vi "CheckColision_1AsterNShoots.vi"(8 "Error In":errorcluster, 9 "ShootsInfo":cluster{"ShootData":T1, "Cluster":T2}[](array[cluster]), 10 "AsterData":T2, 11 "AsterObjectRef":refnum<vi>) -> (0 "Error Out":errorcluster, 1 "ShootsInfoOut":cluster{"ShootData":T1, "Cluster":T2}[](array[cluster]))   [LabVIEW 2017]
uses:
  HoldData/DataForColision.ctl
  ManRef_ShootData.ctl
  Asteroid/Asteroid_states.ctl
  Spaceship/Shoot/Shoot_states.ctl
  HoldData/HoldData_mods.ctl
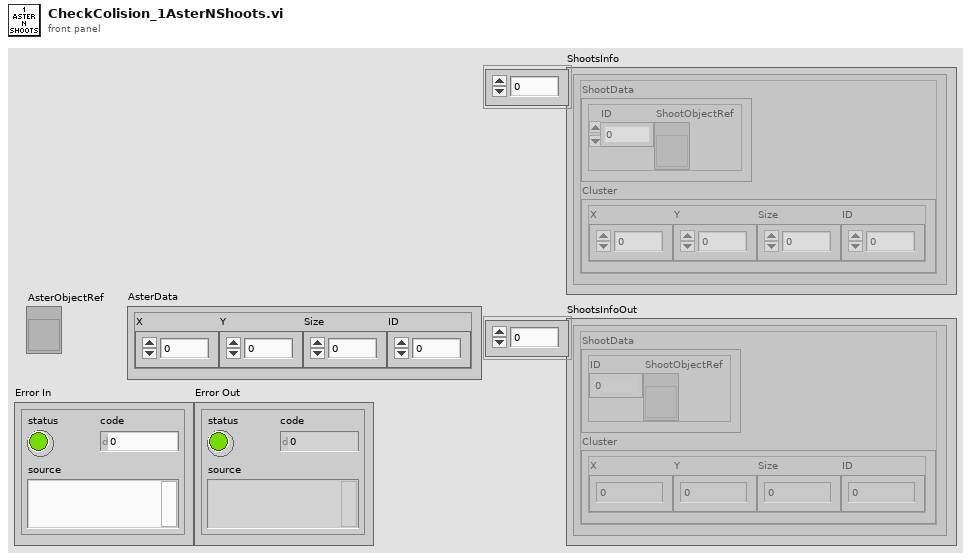
[diagram p1: front panel]
types:
  T1 = typedef "ManRef_ShootData.ctl" = cluster{"ID":i32, "ShootObjectRef":refnum<vi>}
  T2 = typedef "DataForColision.ctl" = cluster{"X":dbl, "Y":dbl, "Size":dbl, "ID":i32}
  T3 = typedef "HoldData_mods.ctl" = enum16{"Init", "NewAster", "UpdateAster", "RemoveAster", "GetAsterData", "NewShoot", "UpdateShoot", "RemoveShoot", "GetShootData", "End"}
  T4 = typedef "Shoot_states.ctl" = enum16{"Init", "Move", "Draw", "Destroy"}
  T5 = typedef "Asteroid_states.ctl" = enum16{"Init", "Move", "Split", "Draw", "Destroy"}
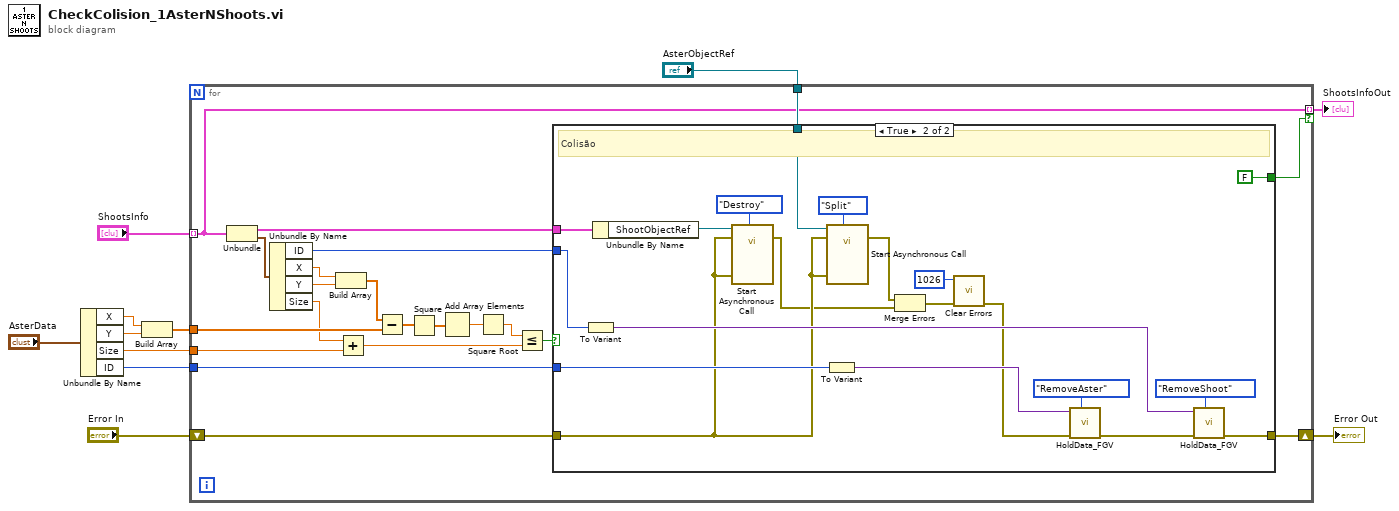
[diagram p0: block diagram]
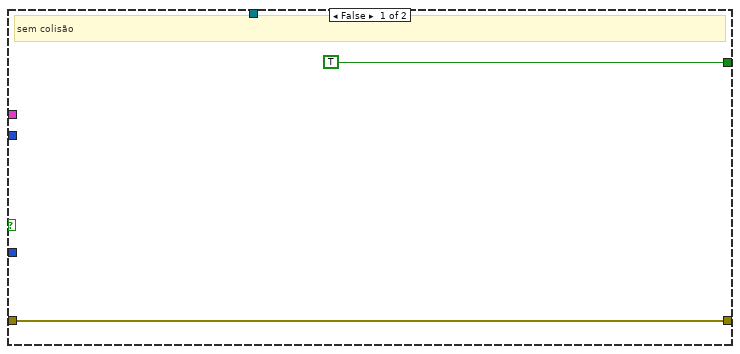
[diagram p2: hidden frame]
diagram:
  n1 = Unbundle By Name("AsterData") -> ("X"=w10:dbl, "Y"=w11:dbl, "Size"=w5:dbl, "ID"=w1:i32)
  n2 = Build Array(w10, w11) -> (w9:dbl[])
  n3 = for {
    tunnel: w5 -> [w16]
    tunnel: w9 -> [w29]
    shift-right: [w22] -> w7
    shift-left: "Error In" -> [w23]
    tunnel: "AsterObjectRef" -> [w21]
    tunnel: "ShootsInfo" -> [w18] mode=indexing
    tunnel: [w18] -> w2 mode=indexing if=w17
    tunnel: w1 -> [w13]
    n4 = Unbundle(w18) -> ("ShootData"=w20:T1, "Cluster"=w19:T2)
    n5 = Unbundle By Name(w19) -> ("ID"=w12:i32, "X"=w32:dbl, "Y"=w31:dbl, "Size"=w15:dbl)
    n6 = Build Array(w32, w31) -> (w30:dbl[])
    n7 = Add(x=w15, y=w16) -> (x+y=w14:dbl)
    n8 = Subtract(x=w30, y=w29) -> (x-y=w28:dbl[])
    n9 = Square(x=w28) -> (x^2=w27:dbl[])
    n10 = Add Array Elements(numeric array=w27) -> (sum=w26:dbl)
    n11 = Square Root(x=w26) -> (sqrt(x)=w25:dbl)
    n12 = Less Or Equal?(x=w25, y=w14) -> (x <= y?=w24:bool)
    n13 = case shown="True" w24 {
      tunnel: w20 -> [_ w54]
      tunnel: w23 -> [w34 w38]
      tunnel: [w34 w42] -> w22
      tunnel: w21 -> [_ w53]
      tunnel: [TRUE FALSE] -> w17
      tunnel: w13 -> [_ w47]
      tunnel: w12 -> [_ w45]
      frame False {
        # "sem colisão"
      }
      frame True {
        # "Colisão"
        n14 = To Variant(anything=w45) -> (Variant=w41:variant)
        n15 = Unbundle By Name(w54) -> ("ShootObjectRef"=w51:refnum<vi>)
        n16 = call-by-ref "Start Asynchronous Call"(reference=w51, error in=w38, "Shoot_states"=Shoot_states."Destroy", "error in"=w38) -> (error out=w37:errorcluster)  [unwired: 9 in, 2 out]
        n17 = call-by-ref "Start Asynchronous Call"(reference=w53, error in=w38, "Asteroid_states"=Asteroid_states."Split", "error in"=w38) -> (error out=w36:errorcluster)  [unwired: 9 in, 2 out]
        n18 = To Variant(anything=w47) -> (Variant=w46:variant)
        n19 = Merge Errors(w36, w37) -> (w35:errorcluster)
        n20 = call <vilib>:"Clear Errors.vi"("error in (no error)"=w35, "specific error code to clear (0: all)"=1026) -> ("error out"=w39:errorcluster)  [unwired: 4 in, 1 out]
        n21 = call "HoldData_FGV.vi"("HoldData_mods"=HoldData_mods."RemoveAster", "error in"=w39, "DataIn"=w46) -> ("error out"=w43:errorcluster)  [unwired: 7 in, 1 out]
        n22 = call "HoldData_FGV.vi"("HoldData_mods"=HoldData_mods."RemoveShoot", "error in"=w43, "DataIn"=w41) -> ("error out"=w42:errorcluster)  [unwired: 7 in, 1 out]
      }
    }
  }
  "Error Out" <- w7
  "ShootsInfoOut" <- w2
